vi "Unregister.vi"(8 "Error In":errorcluster, 10 "Listener ID":string, 11 "Listeners In":refnum<queue>[](array[refnum])) -> (0 "Error Out":errorcluster, 3 "Listeners Out":refnum<queue>[](array[refnum]))   [LabVIEW 2015, in "Logger.lvlib"]
uses:
  Logger.lvlib
  Public/Controls/Message.ctl
  Public/Controls/Tag.ctl
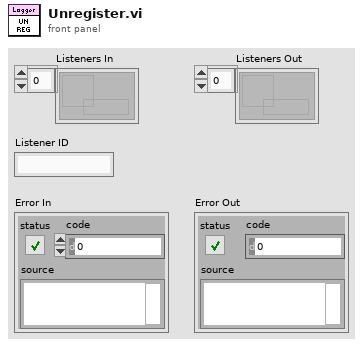
[diagram p1: front panel]
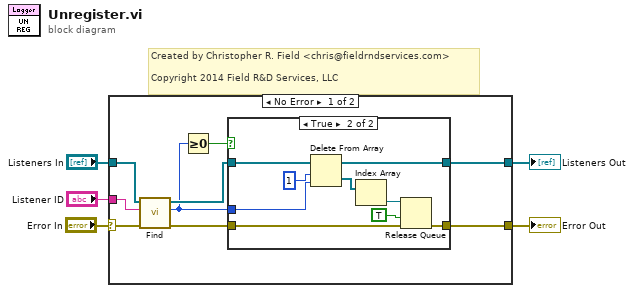
[diagram p0: block diagram]
diagram:
  # "Created by Christopher R. Field <chris@fieldrndservices.com>\n\nCopyright 2014 Field R&D Services, LLC"
  n1 = case shown="No Error" "Error In" {
    selector: "Error In" -> [w7 w26]
    tunnel: [w14 w26] -> w5
    tunnel: [w13 w27] -> w4
    tunnel: "Listeners In" -> [w11 w27]
    tunnel: "Listener ID" -> [w8 _]
    frame No Error {
      n2 = call "Find.vi"("Error In"=w7, "Listener ID"=w8, "Listeners In"=w11) -> ("Error Out"=w6:errorcluster, "Index"=w9:i32, "Listeners Out"=w10:refnum<queue>[])  [unwired: 6 in]
      n3 = Greater Or Equal To 0?(x=w9) -> (x >= 0?=w12:bool)
      n4 = case shown="True" w12 {
        tunnel: w10 -> [w16 w25]
        tunnel: w9 -> [_ w23]
        tunnel: [w16 w22] -> w13
        tunnel: w6 -> [w15 w19]
        tunnel: [w15 w18] -> w14
        frame False {
        }
        frame True {
          n5 = Delete From Array(array=w25, length=1, index=w23) -> (deleted portion=w21:refnum<queue>[], array with subset deleted=w22:refnum<queue>[])
          n6 = Index Array(array=w21) -> (element=w20:refnum<queue>)  [unwired: 1 in]
          n7 = Release Queue(queue=w20, force destroy? (F)=TRUE, error in (no error)=w19) -> (error out=w18:errorcluster)  [unwired: 2 out]
        }
      }
    }
    frame Error {
    }
  }
  "Error Out" <- w5
  "Listeners Out" <- w4
